vi "Probe_Setup_Options.vi"() -> (2 "Probes":string[](array[string]))   [LabVIEW 2022 SP3]
uses:
  <vilib>/Utility/error.llb/Trim Whitespace One-Sided.vi
  Globals/Constants_global.vi
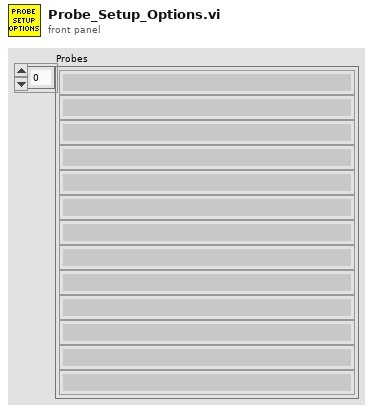
[diagram p1: front panel]
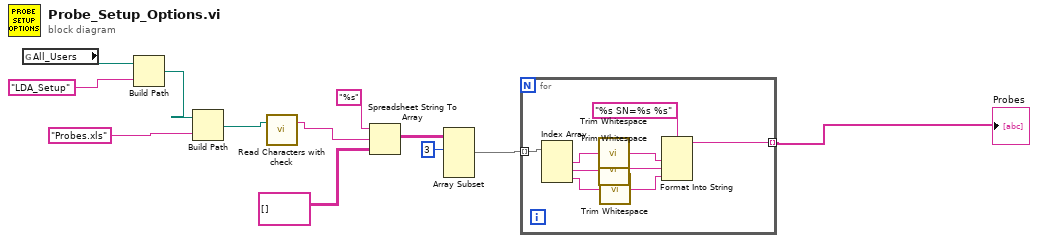
[diagram p0: block diagram]
diagram:
  n1 = global read "Constants_global.vi" "All_Users"() -> (w11:path)
  n2 = Build Path(base path=w11, name or relative path="LDA_Setup") -> (appended path=w10:path)
  n3 = Build Path(base path=w10, name or relative path="Probes.xls") -> (appended path=w2:path)
  n4 = call "Read Characters with check.vi"("file (use dialog)"=w2) -> ("Read String"=w1:string)  [unwired: 1 in, 1 out]
  n5 = Spreadsheet String To Array(format string="%s", spreadsheet string=w1, array type (2D Dbl)=string[][] []) -> (array=w7:string[][])  [unwired: 1 in]
  n6 = Array Subset(array=w7, index (row)=3 ("index")) -> (w3:string[][])  [unwired: 3 in]
  n7 = for {
    tunnel: w3 -> [w21] mode=indexing
    tunnel: [w19] -> w12 mode=indexing
    n8 = Index Array(array=w21) -> (element #1=w18:string, element #2=w16:string, element #3=w14:string)  [unwired: 3 in]
    n9 = call <vilib>:"Trim Whitespace.vi"("string"=w18) -> ("trimmed string"=w17:string)  [unwired: 1 in]
    n10 = call <vilib>:"Trim Whitespace.vi"("string"=w16) -> ("trimmed string"=w15:string)  [unwired: 1 in]
    n11 = call <vilib>:"Trim Whitespace.vi"("string"=w14) -> ("trimmed string"=w13:string)  [unwired: 1 in]
    n12 = Format Into String(format string="%s SN=%s %s", w17, w15, w13) -> (resulting string=w19:string)  [unwired: 2 in, 1 out]
  }
  "Probes" <- w12
